vi "Test Insert.vi"() -> ()   [LabVIEW 2013]
uses:
  ROS/Code/SubVIs/BaxterSide.ctl
  <vilib>/Utility/config.llb/Read Key (String).vi
  Move/Move Axis.vi
  Arm Globals.vi
  <vilib>/Utility/config.llb/NI_LVConfig.lvlib
panel:
  in  "Stop":bool
  out "Status":string
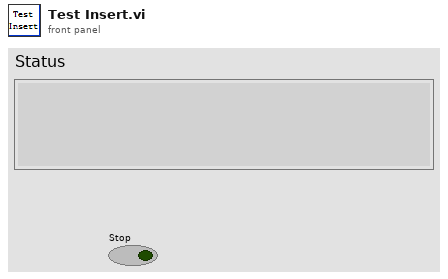
[diagram p1: front panel]
types:
  T1 = typedef "BaxterSide.ctl" = enum16{"left", "right"}
  T2 = typedef "NI_LVConfig.lvlib/Config Data RefNum.ctl" = refnum<k1>
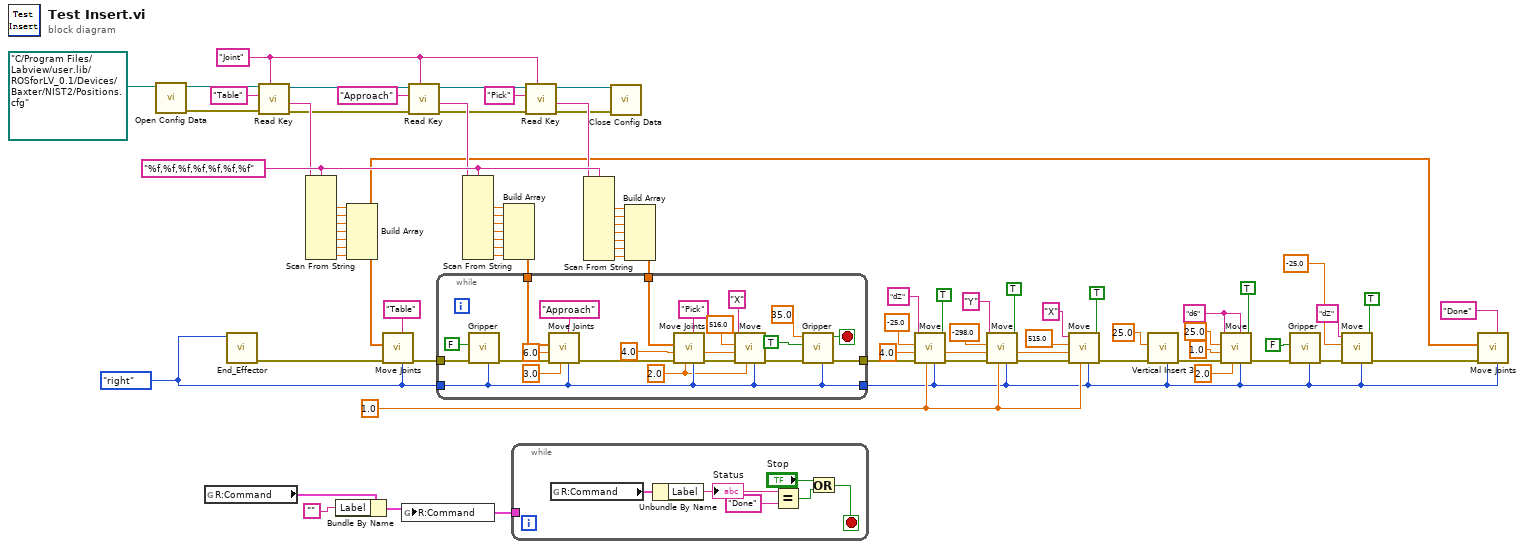
[diagram p0: block diagram]
diagram:
  w12 = "d6" ("Location")
  w13 = 1.0 ("Wait (s)")
  w8 = 4.0 ("Speed (mm/s)")
  w20 = BaxterSide."right" ("Side")
  w48 = "%f,%f,%f,%f,%f,%f,%f" ("format string")
  w72 = "Joint" ("section")
  n1 = call <vilib>:"Open Config Data.vi"("configuration file path"=path "C:/Program Files/Labview/user.lib/ROSforLV_0.1/Devices/Baxter/NIST2/Positions.cfg") -> ("error out"=w75:errorcluster, "refnum"=w77:T2)  [unwired: 8 in, 1 out]
  n2 = global read "Arm Globals.vi" "R:Command"() -> (w28:cluster{"Label":string, "Angles":dbl[]})
  n3 = call "End_Effector.vi"("Side"=w20) -> ("error out"=w38:errorcluster)  [unwired: 7 in]
  n4 = call-poly <vilib>:"Read Key.vi"("section"=w72, "error in (no error)"=w75, "key"="Table", "refnum"=w77) -> ("error out"=w41:errorcluster, "value"=w46:string, "refnum out"=w74:T2)  [unwired: 4 in, 1 out]
  n5 = Scan From String(format string=w48, input string=w46) -> (output 1=w69:dbl, output 2=w68:dbl, output 3=w67:dbl, output 4=w66:dbl, output 5=w65:dbl, output 6=w64:dbl, output 7=w63:dbl)  [unwired: 9 in, 3 out]
  n6 = Bundle By Name(cluster=w28, "Label"="") -> (w26:cluster{"Label":string, "Angles":dbl[]})
  n7 = Build Array(w69, w68, w67, w66, w65, w64, w63) -> (w30:dbl[])
  n8 = call "Move Joints.vi"("Side"=w20, "Label"="Table", "error in"=w38, "Goal"=w30) -> ("error out"=w24:errorcluster)  [unwired: 6 in, 1 out]
  n9 = global write "Arm Globals.vi" "R:Command"(w26) -> ()
  n10 = call-poly <vilib>:"Read Key.vi"("section"=w72, "error in (no error)"=w41, "key"="Approach", "refnum"=w74) -> ("error out"=w42:errorcluster, "value"=w47:string, "refnum out"=w73:T2)  [unwired: 4 in, 1 out]
  n11 = Scan From String(format string=w48, input string=w47) -> (output 1=w62:dbl, output 2=w61:dbl, output 3=w60:dbl, output 4=w59:dbl, output 5=w58:dbl, output 6=w57:dbl, output 7=w56:dbl)  [unwired: 9 in, 3 out]
  n12 = Build Array(w62, w61, w60, w59, w58, w57, w56) -> (w40:dbl[])
  n13 = while {
    tunnel: w26 -> [_]
    stop <- w81 stop-if-true
    n14 = global read "Arm Globals.vi" "R:Command"() -> (w85:cluster{"Label":string, "Angles":dbl[]})
    n15 = Unbundle By Name(w85) -> ("Label"=w84:string)
    "Status" <- w84
    n16 = Equal?(x=w84, y="Done") -> (x = y?=w82:bool)
    n17 = Or(x="Stop", y=w82) -> (x .or. y?=w81:bool)
  }
  n18 = call-poly <vilib>:"Read Key.vi"("section"=w72, "error in (no error)"=w42, "key"="Pick", "refnum"=w73) -> ("error out"=w43:errorcluster, "value"=w45:string, "refnum out"=w44:T2)  [unwired: 4 in, 1 out]
  n19 = Scan From String(format string=w48, input string=w45) -> (output 1=w55:dbl, output 2=w54:dbl, output 3=w53:dbl, output 4=w52:dbl, output 5=w51:dbl, output 6=w50:dbl, output 7=w49:dbl)  [unwired: 9 in, 3 out]
  n20 = call <vilib>:"Close Config Data.vi"("error in (no error)"=w43, "refnum"=w44) -> ()  [unwired: 8 in, 2 out]
  n21 = Build Array(w55, w54, w53, w52, w51, w50, w49) -> (w39:dbl[])
  n22 = while {
    tunnel: w40 -> [w104]
    tunnel: w39 -> [w103]
    tunnel: [w100] -> w25
    tunnel: w24 -> [w97]
    tunnel: w20 -> [w90]
    tunnel: [w90] -> w1
    stop <- w94 stop-if-true
    w86 = 2.0 ("Wait (s)")
    w91 = 4.0 ("time")
    n23 = call "Gripper.vi"("Side"=w90, "error in"=w97, "Open?"=FALSE) -> ("error out"=w96:errorcluster)  [unwired: 7 in, 1 out]
    n24 = call "Move Joints.vi"("Side"=w90, "Label"="Approach", "Wait (s)"=3.0, "error in"=w96, "time"=6.0, "Goal"=w104) -> ("error out"=w87:errorcluster)  [unwired: 4 in, 1 out]
    n25 = call "Move Joints.vi"("Side"=w90, "Label"="Pick", "Wait (s)"=w86, "error in"=w87, "time"=w91, "Goal"=w103) -> ("error out"=w89:errorcluster)  [unwired: 4 in, 1 out]
    n26 = call-poly "Move.vi"("Side"=w90, "Wait Time"=w86, "error in"=w89, "Speed"=w91, "Value"=516.0 ("Speed (mm/s)"), "Location"="X") -> ("error out"=w88:errorcluster)  [unwired: 5 in]
    n27 = call "Gripper.vi"("Side"=w90, "error in"=w88, "Open?"=TRUE ("Close"), "Target Position"=sgl 35.0) -> ("error out"=w100:errorcluster, "On Target"=w94:bool)  [unwired: 6 in]
  }
  n28 = call-poly "Move.vi"("Make Vertical"=TRUE, "Side"=w1, "Wait Time"=w13, "error in"=w25, "Speed"=w8, "Value"=-25.0 ("Speed (mm/s)"), "Location"="dZ") -> ("error out"=w34:errorcluster)  [unwired: 4 in]
  n29 = call-poly "Move.vi"("Make Vertical"=TRUE, "Side"=w1, "Wait Time"=w13, "error in"=w34, "Speed"=w8, "Value"=-298.0 ("Speed (mm/s)"), "Location"="Y") -> ("error out"=w22:errorcluster)  [unwired: 4 in]
  n30 = call-poly "Move.vi"("Make Vertical"=TRUE, "Side"=w1, "Wait Time"=w13, "error in"=w22, "Speed"=w8, "Value"=515.0 ("Speed (mm/s)"), "Location"="X") -> ("error out"=w21:errorcluster)  [unwired: 4 in]
  n31 = call "Vertical Insert 3.vi"("Side"=w1, "error in"=w21, "depth"=25.0) -> ("error out"=w15:errorcluster)  [unwired: 8 in]
  n32 = call-poly "Move.vi"("Make Vertical"=TRUE, "Side"=w1, "Label"=w12, "Wait Time"=2.0, "error in"=w15, "Speed"=1.0, "Value"=25.0 ("depth"), "Location"=w12) -> ("error out"=w14:errorcluster)  [unwired: 3 in]
  n33 = call "Gripper.vi"("Side"=w1, "error in"=w14, "Open?"=FALSE) -> ("error out"=w6:errorcluster)  [unwired: 7 in, 1 out]
  n34 = call-poly "Move.vi"("Make Vertical"=TRUE, "Side"=w1, "error in"=w6, "Value"=-25.0 ("Speed (mm/s)"), "Location"="dZ") -> ("error out"=w5:errorcluster)  [unwired: 6 in]
  n35 = call "Move Joints.vi"("Side"=w1, "Label"="Done", "error in"=w5, "Goal"=w30) -> ()  [unwired: 6 in, 2 out]
